vi "Init Actor Core.vi"(8 "error in (no error)":errorcluster, 11 "Measure Object in":refnum<class "Measure App.lvclass">) -> (0 "error out":errorcluster, 3 "Measure Object out":refnum<class "Measure App.lvclass">)   [LabVIEW 2016, in "Measure App.lvclass"]
uses:
  Measure App.lvclass
  Controllers/Sequence Controller/Sequence Controller.lvclass
  C:/github/LabActor/Worker/Worker.lvclass
  Measure App.lvclass/Measure App.ctl
  Template Module Messages/Attach to Sub-pannel Msg/Attach to Sub-pannel Msg.lvclass/Attach to Sub-pannel Msg.ctl
  <vilib>/ActorFramework/Message Enqueuer/Message Enqueuer.lvclass/Message Enqueuer.ctl
  <vilib>/ActorFramework/Message Enqueuer/Enqueue.vi
  Template Module Messages/Attach to Sub-pannel Msg/Attach to Sub-pannel Msg.lvclass
  C:/Program Files (x86)/National Instruments/LabVIEW 2016/vi.lib/ActorFramework/Message/Message.lvclass
  <vilib>/ActorFramework/Message Priority Queue/Priority Enqueue.vi
  Controllers/Application Controller/Application Controller.lvclass
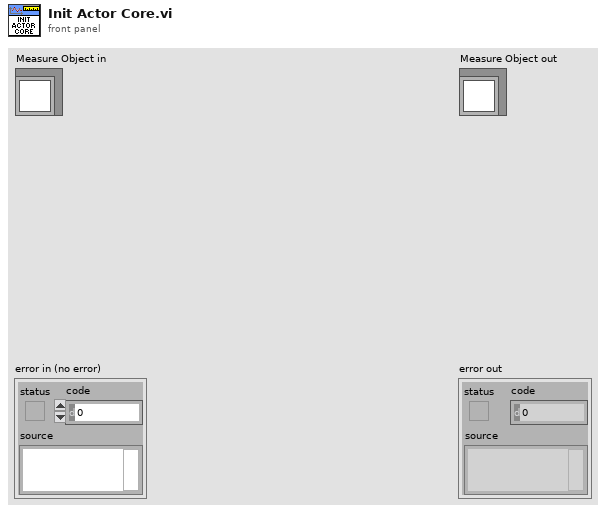
[diagram p1: front panel]
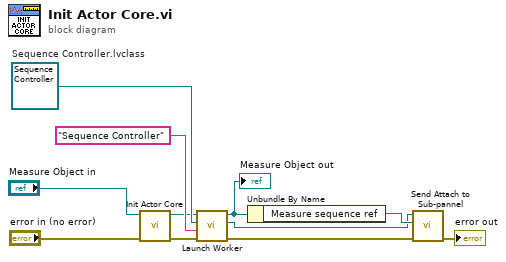
[diagram p0: block diagram]
diagram:
  w9 = refnum<class "Sequence Controller.lvclass"> refnum  # Sequence Controller.lvclass
  n1 = call-parent "Init Actor Core.vi"("error in (no error)"="error in (no error)", "Measure Object in"="Measure Object in") -> ("error out"=w7:errorcluster, "Measure Object out"=w6:refnum<class "Measure App.lvclass">)  [unwired: 8 in]
  n2 = call-dynamic "Launch Worker.vi"("error in (no error)"=w7, "Name"="Sequence Controller", "Subordinate Object"=w9, "Application Controller in"=w6) -> ("error out"=w2:errorcluster, "Nested Actor's Enqueuer"=w3:refnum<class "Message Enqueuer.lvclass">, "Application Controller out"=w5:refnum<class "Measure App.lvclass">)  [unwired: 5 in]
  "Measure Object out" <- w5
  n3 = Unbundle By Name(w5) -> ("Measure sequence ref"=w4:refnum<vi>)
  n4 = call "Send Attach to Sub-pannel.vi"("error in (no error)"=w2, "Sub-pannel ref"=w4, "Message Enqueuer"=w3) -> ("error out"=→"error out":errorcluster)  [unwired: 7 in, 1 out]
